vi "ATF Storage-Data Transfer Loop RD.vi"(11 "Data FIFO Ref":T1) -> ()   [LabVIEW 2022 SP3]
uses:
  RT Controls/ATF Storage-Data FIFO.ctl
  RT Controls/ATF Storage-DiplayPC comm ctrl.ctl
  <vilib>/Platform/TimedLoop/XDataNode/timing_clust.ctl
  <vilib>/Platform/TimedLoop/XDataNode/nitl_modes.ctl
  <vilib>/Platform/TimedLoop/XDataNode/wakeup.ctl
  RT Support/ATF Storage-RT_Global_R.vi
  <vilib>/platform/TimedLoop/XDataNode/XDataNode.xnode
  <vilib>/Platform/TimedLoop/XDataNode/XDNodeRunTimeDep.lvlib
panel:
  out "x-y":u32
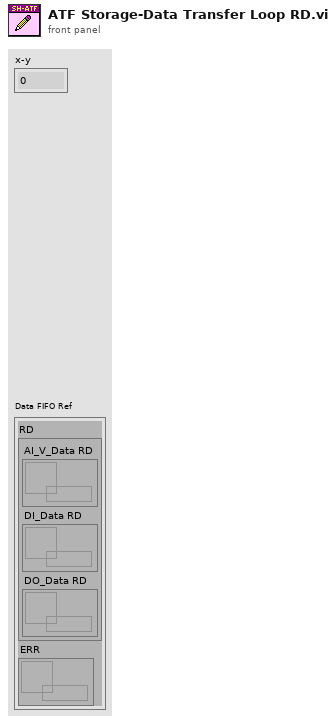
[diagram p1: front panel]
types:
  T1 = typedef "ATF Storage-Data FIFO.ctl" = cluster{"RD":cluster{"AI_V_Data RD":refnum<queue>, "DI_Data RD":refnum<queue>, "DO_Data RD":refnum<queue>}, "ERR":refnum<queue>}
  T2 = typedef "ATF Storage-DiplayPC comm ctrl.ctl" = enum16{"Initialize", "Listen for UI Writer", "Send RT Data"}
  T3 = typedef "XDNodeRunTimeDep.lvlib/timing_clust.ctl" = cluster{"Expected End [f-1]":u64, "Actual End [f-1]":u64, "Finished Late? [f-1]":bool, "Expected End [i-1]":u64, "Actual End [i-1]":u64, "Finished Late? [i-1]":bool, "Expected Start [i]":u64, "Actual Start [i]":u64, "Expected Start [f]":u64, "Actual Start [f]":u64, "Source Name":string, "Structure Name":string, "Period":i64, "Deadline":i64, "Offset":i64, "Start":i64, "Priority":i32, "Timeout":i32, "Mode":T4, "Wakeup Reason":T5, "Error":errorcluster, "Source Type":string, "Secondary Source Type":string, "Global End Time":u64, "Global Start Time":u64, "Frame Duration":u64, "Iteration Duration":u64, "Assigned CPU":i32, "I/O Scan Engine Mode":u32}
  T4 = typedef "XDNodeRunTimeDep.lvlib/nitl_modes.ctl" = enum32{"No Change", "Process missed periods, maintain original phase", "Discard missed periods, maintain original phase", "Process missed periods, ignore original phase", "Discard missed periods, ignore original phase"}
  T5 = typedef "XDNodeRunTimeDep.lvlib/wakeup.ctl" = enum32{"Normal", "Aborted", "Asynchronous wakeup", "Timing source error", "Timed loop error", "Timeout"}
  T6 = cluster{"Start DAQ":bool, "Stop DAQ":bool, "RT Stop":bool, "RT Exit":bool, "Start Seq":bool}
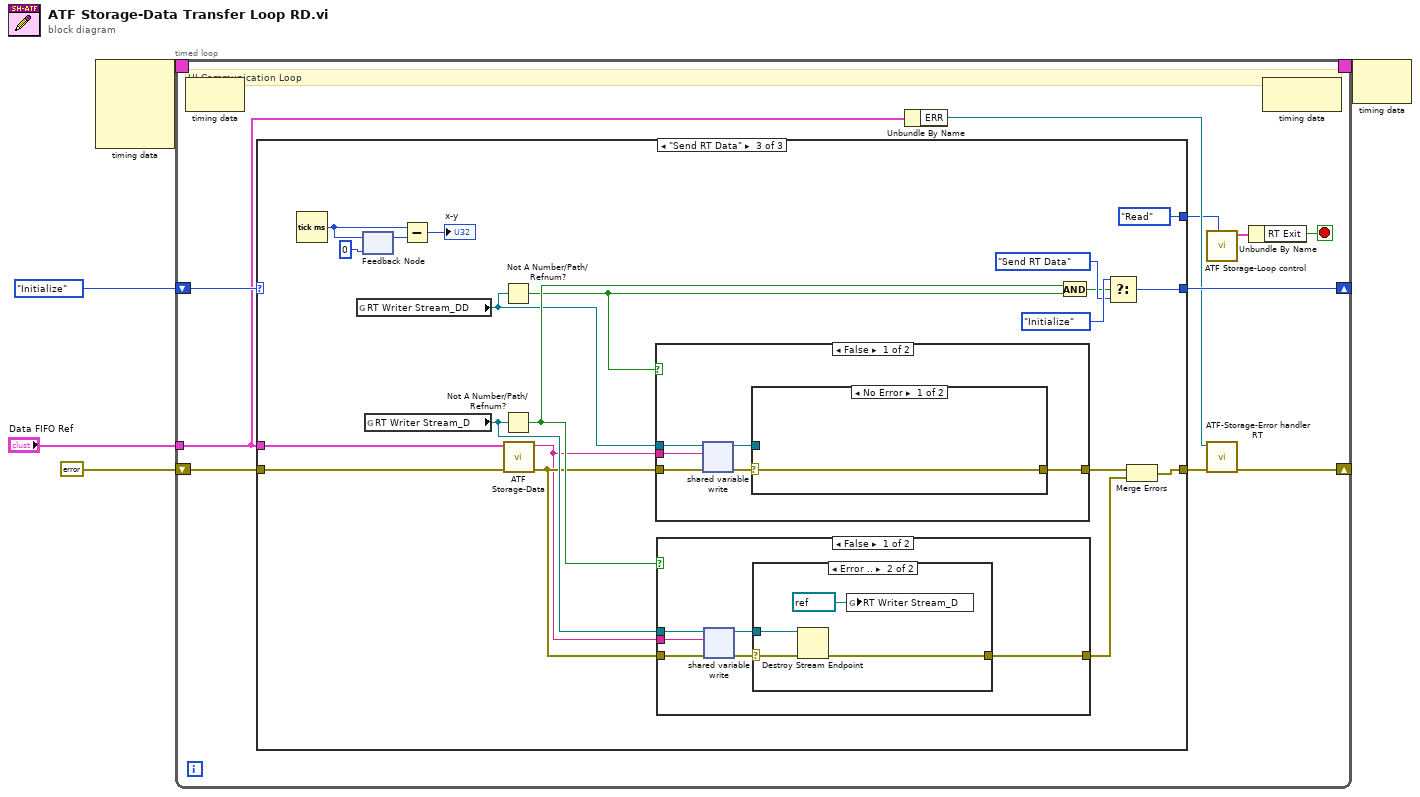
[diagram p0: block diagram]
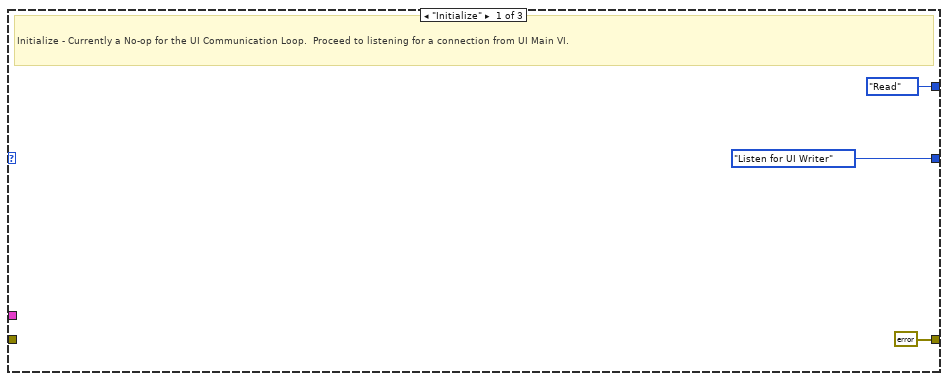
[diagram p2: hidden frame]
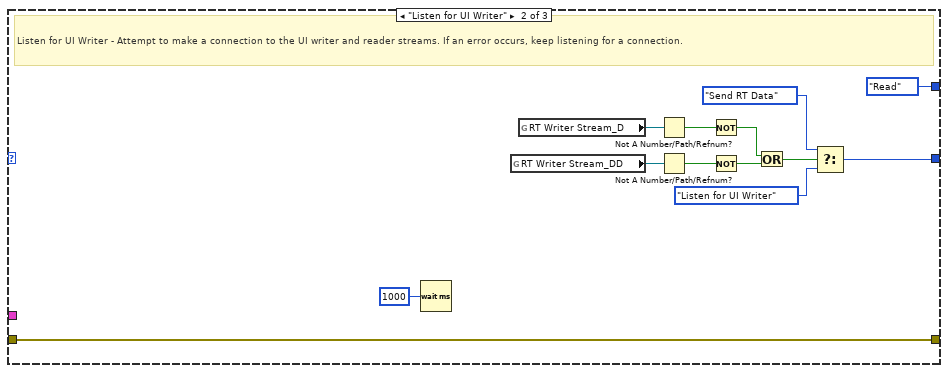
[diagram p3: hidden frame]
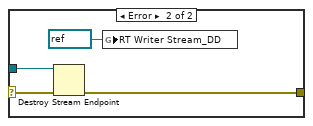
[diagram p4: hidden frame]
diagram:
  n1 = node-c288() -> (w2:T3)  [unwired: 4 in]
  n2 = timed-loop {
    shift-right: [w15] -> _
    shift-left: ATF_Storage-DiplayPC_comm_ctrl."Initialize" -> [w14]
    tunnel: "Data FIFO Ref" -> [w9]
    shift-right: [w6] -> _
    shift-left: errorcluster {"status"=FALSE, "code"=0, "source"=""} ("error in (no error)") -> [w10]
    timing: w2 -> [_]
    timing-out: [_] -> w1
    stop <- w12 stop-if-true
    # "UI Communication Loop"
    n3 = node-c288() -> ()  [unwired: 1 in, 1 out]
    n4 = case shown="\"Send RT Data\"" w14 {
      tunnel: [errorcluster {"status"=FALSE, "code"=0, "source"=""} ("error IO") w22 w38] -> w11
      tunnel: [ATF_Storage-DiplayPC_comm_ctrl."Listen for UI Writer" w27 w49] -> w15
      tunnel: w9 -> [_ _ w40]
      tunnel: w10 -> [_ w22 w41]
      tunnel: [enum16{"Init", "Write", "Read"}."Read" ("Action") enum16{"Init", "Write", "Read"}."Read" ("Action") enum16{"Init", "Write", "Read"}."Read" ("Action")] -> w7
      frame "Initialize" {
        # "Initialize - Currently a No-op for the UI Communication Loop.  Proceed to listening for a connection from UI Main VI."
      }
      frame "Listen for UI Writer" {
        # "Listen for UI Writer - Attempt to make a connection to the UI writer and reader streams. If an error occurs, keep listening for a connection."
        n5 = Wait (ms)(milliseconds to wait=u32 1000) -> ()  [unwired: 1 out]
        n6 = global read "ATF Storage-RT_Global_R.vi" "RT Writer Stream_DD"() -> (w32:refnum<k21>)
        n7 = global read "ATF Storage-RT_Global_R.vi" "RT Writer Stream_D"() -> (w33:refnum<k21>)
        n8 = Not A Number/Path/Refnum?(number/path/refnum=w33) -> (NaN/Path/Refnum?=w31:bool)
        n9 = Not A Number/Path/Refnum?(number/path/refnum=w32) -> (NaN/Path/Refnum?=w30:bool)
        n10 = Not(x=w31) -> (.not. x?=w29:bool)
        n11 = Not(x=w30) -> (.not. x?=w28:bool)
        n12 = Or(x=w29, y=w28) -> (x .or. y?=w24:bool)
        n13 = Select(t=ATF_Storage-DiplayPC_comm_ctrl."Send RT Data", s=w24, f=ATF_Storage-DiplayPC_comm_ctrl."Listen for UI Writer") -> (s? t:f=w27:T2)
      }
      frame "Send RT Data" {
        n14 = Tick Count (ms)() -> (millisecond timer value=w46:u32)
        n15 = global read "ATF Storage-RT_Global_R.vi" "RT Writer Stream_DD"() -> (w47:refnum<k21>)
        n16 = feedback-in #1(w46) -> ()
        n17 = feedback #1(u32 0 ("millisecond timer value")) -> (w45:u32)
        n18 = global read "ATF Storage-RT_Global_R.vi" "RT Writer Stream_D"() -> (w53:refnum<k21>)
        n19 = Subtract(x=w46, y=w45) -> (x-y=→"x-y":u32)
        n20 = Not A Number/Path/Refnum?(number/path/refnum=w47) -> (NaN/Path/Refnum?=w42:bool)
        n21 = Not A Number/Path/Refnum?(number/path/refnum=w53) -> (NaN/Path/Refnum?=w48:bool)
        n22 = call "ATF Storage-Data.vi"("error in (no error)"=w41, "Data FIFO Ref"=w40) -> ("error out"=w36:errorcluster, "data"=w35:string)  [unwired: 8 in]
        n23 = case shown="False" w42 {
          tunnel: w47 -> [w54 _]
          tunnel: w36 -> [w57 w65]
          tunnel: [w56 w65] -> w43
          tunnel: w35 -> [w55 _]
          frame False {
            n24 = shared-variable-write(w54, w57, w55) -> (w58:refnum<k21>, w59:errorcluster)  [unwired: 1 in, 1 out]
            n25 = case shown="No Error" w59 {
              selector: w59 -> [w60 w63]
              tunnel: w58 -> [_ w64]
              tunnel: [w60 w61] -> w56
              frame No Error {
              }
              frame Error {
                n26 = Destroy Stream Endpoint(8:w63, 11:w64) -> (0:w61:errorcluster)
                n27 = global write "ATF Storage-RT_Global_R.vi" "RT Writer Stream_DD"(refnum<k21> refnum ("RT Writer Stream_DD")) -> ()
              }
            }
          }
          frame True {
          }
        }
        n28 = case shown="False" w48 {
          tunnel: w53 -> [w66 _]
          tunnel: w36 -> [w68 w77]
          tunnel: [w69 w77] -> w37
          tunnel: w35 -> [w67 _]
          frame False {
            n29 = shared-variable-write(w66, w68, w67) -> (w70:refnum<k21>, w71:errorcluster)  [unwired: 1 in, 1 out]
            n30 = case shown="Error .." w71 {
              selector: w71 -> [w72 w75]
              tunnel: w70 -> [_ w76]
              tunnel: [w72 w73] -> w69
              frame No Error {
              }
              frame Error {
                n31 = Destroy Stream Endpoint(8:w75, 11:w76) -> (0:w73:errorcluster)
                n32 = global write "ATF Storage-RT_Global_R.vi" "RT Writer Stream_D"(refnum<k21> refnum ("RT Writer Stream_DD")) -> ()
              }
            }
          }
          frame True {
          }
        }
        n33 = And(x=w48, y=w42) -> (x .and. y?=w50:bool)
        n34 = Select(t=ATF_Storage-DiplayPC_comm_ctrl."Initialize", s=w50, f=ATF_Storage-DiplayPC_comm_ctrl."Send RT Data") -> (s? t:f=w49:T2)
        n35 = Merge Errors(w43, w37) -> (w38:errorcluster)
      }
    }
    n36 = Unbundle By Name(w9) -> ("ERR"=w8:refnum<queue>)
    n37 = call "ATF Storage-Loop control.vi"("Action"=w7) -> ("Loop Control out"=w13:T6)  [unwired: 9 in, 1 out]
    n38 = call "ATF-Storage-Error handler RT.vi"("error in"=w11, "Message Queue"=w8) -> ("error out"=w6:errorcluster)  [unwired: 8 in, 1 out]
    n39 = Unbundle By Name(w13) -> ("RT Exit"=w12:bool)
    n40 = node-c288() -> ()  [unwired: 1 in, 1 out]
  }
  n41 = node-c288(w1) -> ()  [unwired: 1 out]
